vi "Get Path Regex.vi"(8 "error in (no error)":errorcluster, 11 "ToggleMuteController in":refnum<class "ToggleMuteController.lvclass">) -> (0 "error out":errorcluster, 2 "Path Regex":string, 3 "ToggleMuteController out":refnum<class "ToggleMuteController.lvclass">)   [LabVIEW 2022 SP3, in "VMR-Deck.lvlib" / "ToggleMuteController.lvclass"]
uses:
  ToggleMuteController.lvclass
  ToggleMuteController.lvclass/ToggleMuteController.ctl
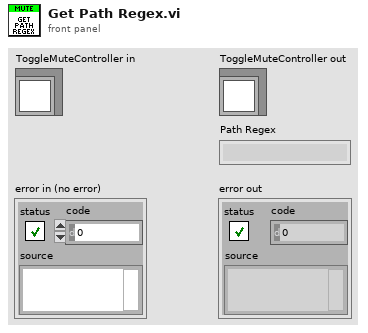
[diagram p1: front panel]
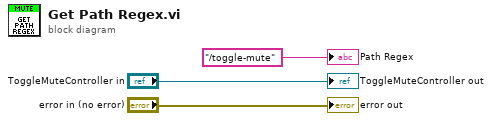
[diagram p0: block diagram]
diagram:
  "error out" <- "error in (no error)"
  "ToggleMuteController out" <- "ToggleMuteController in"
  "Path Regex" <- "/toggle-mute" ("Path Regex")
